vi "Day 6-2.vi"() -> ()   [LabVIEW 2019, in "Day 6.lvlib"]
uses:
  Day 6.lvlib
panel:
  out "Number of days":u64
  out "Final number fo fishes":i32
  out "array":u8[](array[numeric])
  in  "String":string="3,5,1,2,5,4,1,5,1,2,5,5,1,3,1,5,1,3,2,1,5,1,1,1,2,3,1,3,1,2,1,1,5,1,5,4,5,5,3,3,1,5,1,1,5,5,1,3,5,5,3,2,2,4,1,5,3,4,2,5,4,1,2,2,5,1,1,2,4,4,1,3,1,3,1,1,2,2,1,1,5,1,1,4,4,5,5,1,2,1,4,1,1,4,4,3,4,2,2,3,3,2,1,3,3,2,1,1,1,2,1,4,2,2,1,5,5,3,4,5,5,2,5,2,2,5,3,3,1,2,4,2,1,5,1,1,2,3,5,5,1,1,5,5,1,4,5,3,5,2,3,2,4,3,1,4,2,5,1,3,2,1,1,3,4,2,1,1,1,1,2,1,4,3,1,3,1,2,4,1,2,4,3,2,3,5,5,3,3,1,2,3,4,5,2,4,5,1,1,1,4,5,3,5,3,5,1,1,5,1,5,3,1,2,3,4,1,1,4,1,2,4,1,5,4,1,5,4,2,1,5,2,1,3,5,5,4,5,5,1,1,4,1,2,3,5,3,3,1,1,1,4,3,1,1,4,1,5,3,5,1,4,2,5,1,1,4,4,4,2,5,1,2,5,2,1,3,1,5,1,2,1,1,5,2,4,2,1,3,5,5,4,1,1,1,5,5,2,1,1"
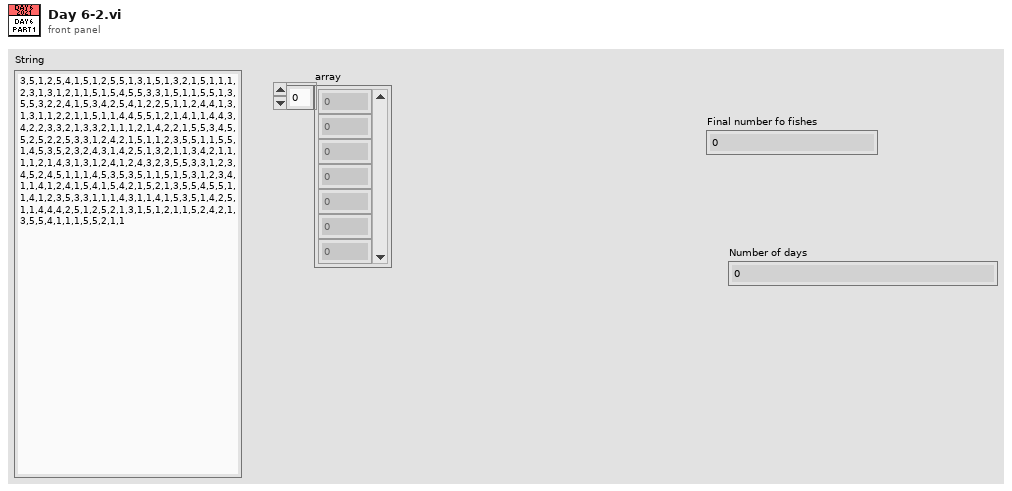
[diagram p1: front panel]
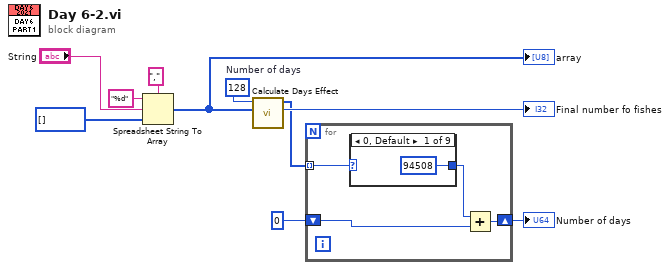
[diagram p0: block diagram]
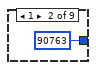
[diagram p2: hidden frame]
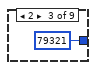
[diagram p3: hidden frame]
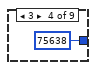
[diagram p4: hidden frame]
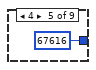
[diagram p5: hidden frame]
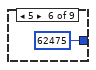
[diagram p6: hidden frame]
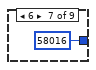
[diagram p7: hidden frame]
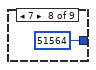
[diagram p8: hidden frame]
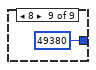
[diagram p9: hidden frame]
diagram:
  w5 = 128  # Number of days
  n1 = Spreadsheet String To Array(delimiter (Tab)=",", format string="%d", spreadsheet string="String", array type (2D Dbl)=u8[] []) -> (array=w6:u8[])
  "array" <- w6
  n2 = call "Calculate Days Effect.vi"("array type (2D Dbl) in"=w6, "Number of days"=w5) -> ("Population size"=→"Final number fo fishes":i32, "array type (2D Dbl) out"=w3:u8[])  [unwired: 8 in]
  n3 = for {
    tunnel: w3 -> [w12] mode=indexing
    shift-right: [w13] -> w1
    shift-left: u64 0 ("Number of days") -> [w14]
    n4 = case shown="0, Default" w12 {
      tunnel: [u64 94508 ("Number of days") u64 90763 ("Number of days") u64 79321 ("Number of days") u64 75638 ("Number of days") u64 67616 ("Number of days") u64 62475 ("Number of days") u64 58016 ("Number of days") u64 51564 ("Number of days") u64 49380 ("Number of days")] -> w11
      frame 0, Default {
      }
      frame 1 {
      }
      frame 2 {
      }
      frame 3 {
      }
      frame 4 {
      }
      frame 5 {
      }
      frame 6 {
      }
      frame 7 {
      }
      frame 8 {
      }
    }
    n5 = Add(x=w11, y=w14) -> (x+y=w13:u64)
  }
  "Number of days" <- w1
